vi "Go To Starting.vi"(8 "error in (no error)":errorcluster, 11 "Command in":refnum<class "Command State Actor.lvclass">) -> (0 "error out":errorcluster, 3 "State out":refnum<class "State Actor.lvclass">)   [LabVIEW 2013, in "Command State Actor.lvlib" / "Command State Actor.lvclass"]
uses:
  Command State Actor.lvclass
  <vilib>/ni/Actors/State Actor/State Actor/State Actor.lvclass
  States/Starting/Starting.lvclass
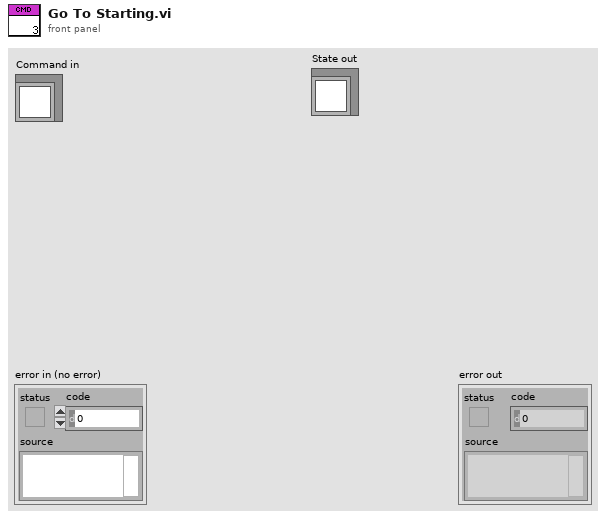
[diagram p1: front panel]
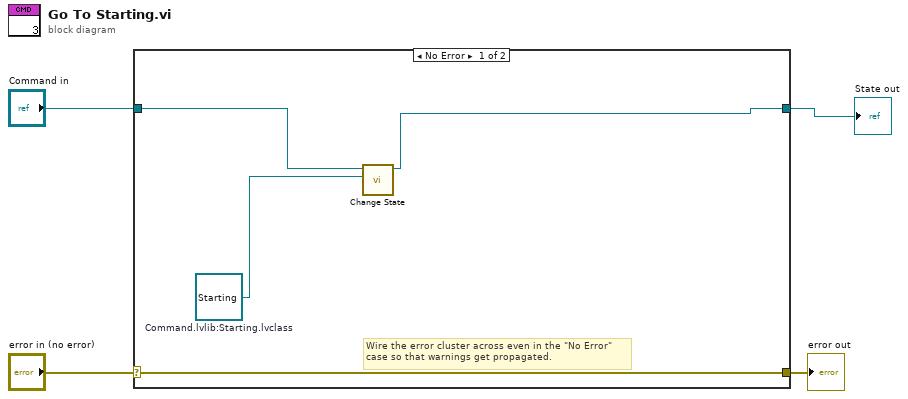
[diagram p0: block diagram]
diagram:
  n1 = case shown="No Error" "error in (no error)" {
    selector: "error in (no error)" -> [w8 w10]
    tunnel: [w8 w10] -> w3
    tunnel: [w6 w9] -> w1
    tunnel: "Command in" -> [w5 w9]
    frame No Error {
      w7 = refnum<class "Starting.lvclass"> refnum  # Command.lvlib:Starting.lvclass
      # "Wire the error cluster across even in the \"No Error\"\ncase so that warnings get propagated."
      n2 = call <vilib>:"Change State.vi"("New State in"=w7, "State in"=w5) -> ("State out"=w6:refnum<class "State Actor.lvclass">)  [unwired: 8 in, 1 out]
    }
    frame Error {
    }
  }
  "error out" <- w3
  "State out" <- w1
